vi "Get Measurement Count.vi"(8 "error in (no error)":errorcluster, 11 "VISA resource name":refnum<visa-resource-name>) -> (0 "error out":errorcluster, 2 "Measurement Count":i32, 3 "VISA resource name out":refnum<visa-resource-name>)   [LabVIEW 2021, in "Keithley 2450.lvlib"]
doc: "This gets the number of measurements to be performed when a measurement is requested."
uses:
  <instrlib>/Keithley 2450/Keithley 2450.lvlib
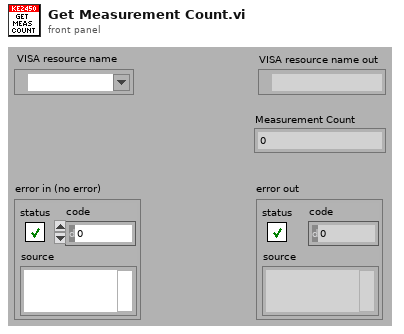
[diagram p1: front panel]
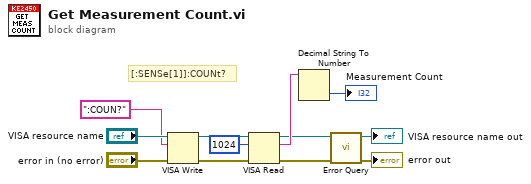
[diagram p0: block diagram]
diagram:
  # "[:SENSe[1]]:COUNt?"
  n1 = VISA Write(VISA resource name="VISA resource name", write buffer=":COUN?", error in (no error)="error in (no error)") -> (VISA resource name out=w11:refnum<visa-resource-name>, error out=w12:errorcluster)  [unwired: 1 out]
  n2 = VISA Read(VISA resource name=w11, byte count=u32 1024, error in (no error)=w12) -> (VISA resource name out=w4:refnum<visa-resource-name>, read buffer=w5:string, error out=w3:errorcluster)  [unwired: 1 out]
  n3 = Decimal String To Number(string=w5) -> (number=→"Measurement Count":i32)  [unwired: 2 in, 1 out]
  n4 = call <instrlib>:"Error Query.vi"("error in (no error)"=w3, "VISA resource name"=w4) -> ("error out"=→"error out":errorcluster, "VISA resource name out"=→"VISA resource name out":refnum<visa-resource-name>)  [unwired: 8 out]
